vi "Read Flow Control Settings.vi"(11 "IActuator in":refnum<class "IActuator.lvclass">) -> (2 "Flow Control Settings":T1={"DAC Channel"=1, "ROT Bias"=70, "Minimum Voltage"=0.0, "Maximum Voltage"=4.096, "Off Value"=0.0} {"Off Value" format="%.3f"; "Maximum Voltage" format="%.3f"; "Minimum Voltage" format="%.3f"; "ROT Bias" max=127 step=1; "DAC Channel" min=1 max=4 step=1}, 3 "IActuator out":refnum<class "IActuator.lvclass">)   [LabVIEW 2015, in "IActuator.lvclass"]
uses:
  IActuator.lvclass
  Typedefs/Flow Control Settings.ctl
  IActuator.lvclass/IActuator.ctl
  Typedefs/FAMTTypedefs.lvlib
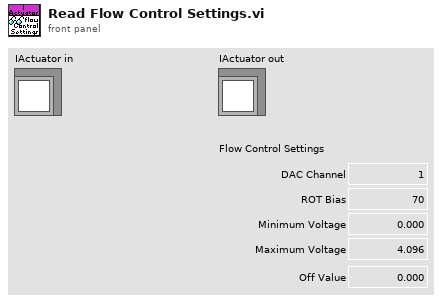
[diagram p1: front panel]
types:
  T1 = typedef "FAMTTypedefs.lvlib/Flow Control Settings.ctl" = cluster{"DAC Channel":u8, "ROT Bias":u8, "Minimum Voltage":dbl, "Maximum Voltage":dbl, "Off Value":dbl}
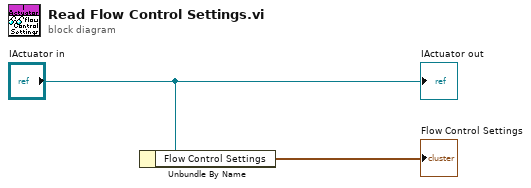
[diagram p0: block diagram]
diagram:
  n1 = Unbundle By Name("IActuator in") -> ("Flow Control Settings"=→"Flow Control Settings":T1)
  "IActuator out" <- "IActuator in"
